vi "Get Schedule.vi"(8 "error in (no error)":errorcluster, 11 "Sequence of SBlocks in":refnum<class "Sequence of SBlocks.lvclass">) -> (0 "error out":errorcluster, 2 "Schedule":refnum<class "Schedule.lvclass">, 3 "Sequence of SBlocks out":refnum<class "Sequence of SBlocks.lvclass">)   [LabVIEW 2020, in "Run Utilities.lvlib" / "Sequence of SBlocks.lvclass"]
uses:
  Sequence of SBlocks.lvclass
  Schedule/Schedule.lvclass
  Sequence of SBlocks.lvclass/Sequence of SBlocks.ctl
  Ancestor/Ancestor/Ancestor.lvclass/Ancestor.ctl
  Support VIs/Generate Error.vi
  FGV/Error Memory/Get Error Description.vi
  Support VIs/Get PC name.vi
  Ancestor/Ancestor/Read ID.vi
  Support VIs/Get Class Name.vi
  <vilib>/Utility/error.llb/Clear Errors.vi
  FGV/Error Memory/Error Memory Core.vi
  <vilib>/AdvancedString/Delimited String to 1D String Array.vi
  Support VIs/Circus Root Path.vi
  FGV/Error Memory/Error Crt Lvl checker.vi
  FGV/Error Memory/Error Memory Core.vi/40c8088d-b597-4017-91af-faa98e00292e.vi
  FGV/Error Memory/Error Memory Core.vi/d4a3ab98-063c-4e44-b43d-fbdcfe6c2be2.vi
  Support VIs/Global Memory.vi
  <vilib>/Utility/LVClass/Get LV Class Name.vi
  Support VIs/Is in Packed Library.vi
  Support VIs/TALOS Root path.vi
  Support VIs/Read CSV worksheet.vi
  Support VIs/Global Constants.vi
  <vilib>/Utility/error.llb/General Error Handler.vi
  Support VIs/Error Log.vi
  Ancestor/Ancestor/Ancestor.lvclass
  <vilib>/Comparison/Equal/Equal Functor/Equal Functor.lvclass
  Schedule Block/Schedule Block.lvclass
  TALOS.lvlib
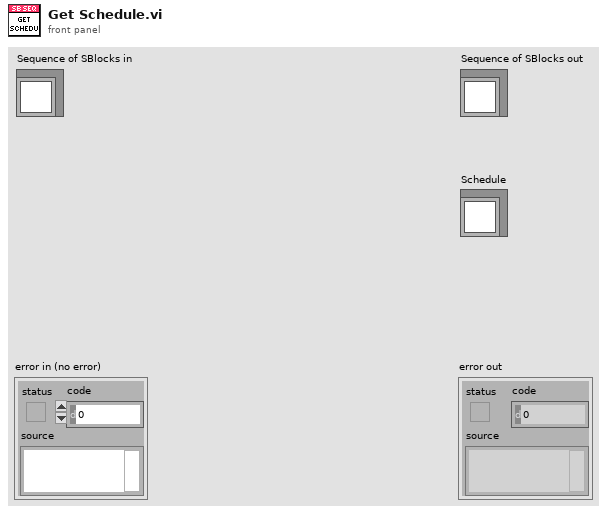
[diagram p1: front panel]
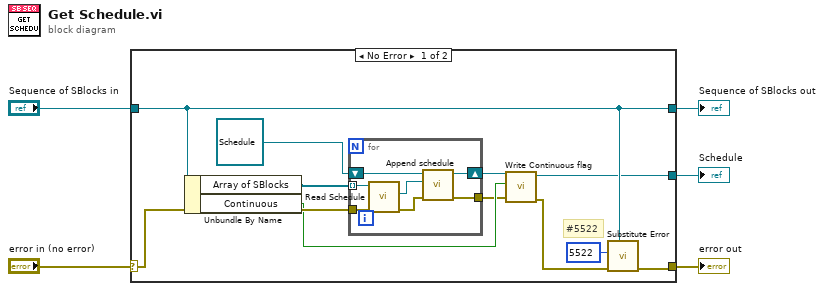
[diagram p0: block diagram]
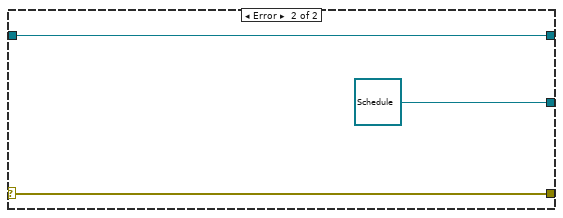
[diagram p2: hidden frame]
diagram:
  n1 = case shown="No Error" "error in (no error)" {
    selector: "error in (no error)" -> [w14 w26]
    tunnel: [w13 w26] -> w4
    tunnel: [w12 w25] -> w2
    tunnel: "Sequence of SBlocks in" -> [w12 w25]
    tunnel: [w9 refnum<class "Schedule.lvclass"> refnum ("Schedule in")] -> w1
    frame No Error {
      # "#5522"
      n2 = Unbundle By Name(w12) -> ("Array of SBlocks"=w16:refnum<class "Schedule Block.lvclass">[], "Continuous"=w8:bool)
      n3 = for {
        tunnel: w16 -> [w19] mode=indexing
        shift-right: [w22] -> w10
        shift-left: refnum<class "Schedule.lvclass"> refnum ("Schedule in") -> [w23]
        tunnel: w14 -> [w20]
        tunnel: [w21] -> w7
        n4 = call-dynamic "Read Schedule.vi"("error in (no error)"=w20, "Schedule Block in"=w19) -> ("error out"=w18:errorcluster, "Schedule"=w17:refnum<class "Schedule.lvclass">)  [unwired: 7 in, 1 out]
        n5 = call-dynamic "Append schedule.vi"("error in (no error)"=w18, "Schedule to append"=w17, "Schedule in"=w23) -> ("error out"=w21:errorcluster, "Schedule out"=w22:refnum<class "Schedule.lvclass">)  [unwired: 7 in]
      }
      n6 = call-dynamic "Write Continuous flag.vi"("error in (no error)"=w7, "Continuous flag"=w8, "Schedule in"=w10) -> ("error out"=w6:errorcluster, "Schedule out"=w9:refnum<class "Schedule.lvclass">)  [unwired: 7 in]
      n7 = call "Substitute Error.vi"("LabVIEW Object"=w12, "error in (no error)"=w6, "Error Code"=5522) -> ("error out"=w13:errorcluster)  [unwired: 8 in]
    }
    frame Error {
    }
  }
  "error out" <- w4
  "Sequence of SBlocks out" <- w2
  "Schedule" <- w1
